vi "ESN_OnlineTraining.vi"(7 "Settings":cluster{"lamda":dbl, "Delta":dbl}={"lamda"=0.995, "Delta"=0.001}, 8 "error in (no error)":errorcluster, 9 "Desired Y(n+1)":dbl[](array[numeric]), 10 "input U(n+1)":dbl[](array[numeric]), 11 "ESN Status":T1) -> (0 "error out":errorcluster, 3 "ESN trained":T1)   [LabVIEW 2010]
uses:
  ESN_Network.ctl
  <vilib>/Analysis/Matrix/Datatypes/RealMatrix.ctl
  <vilib>/Analysis/Matrix/NI_Matrix.lvlib
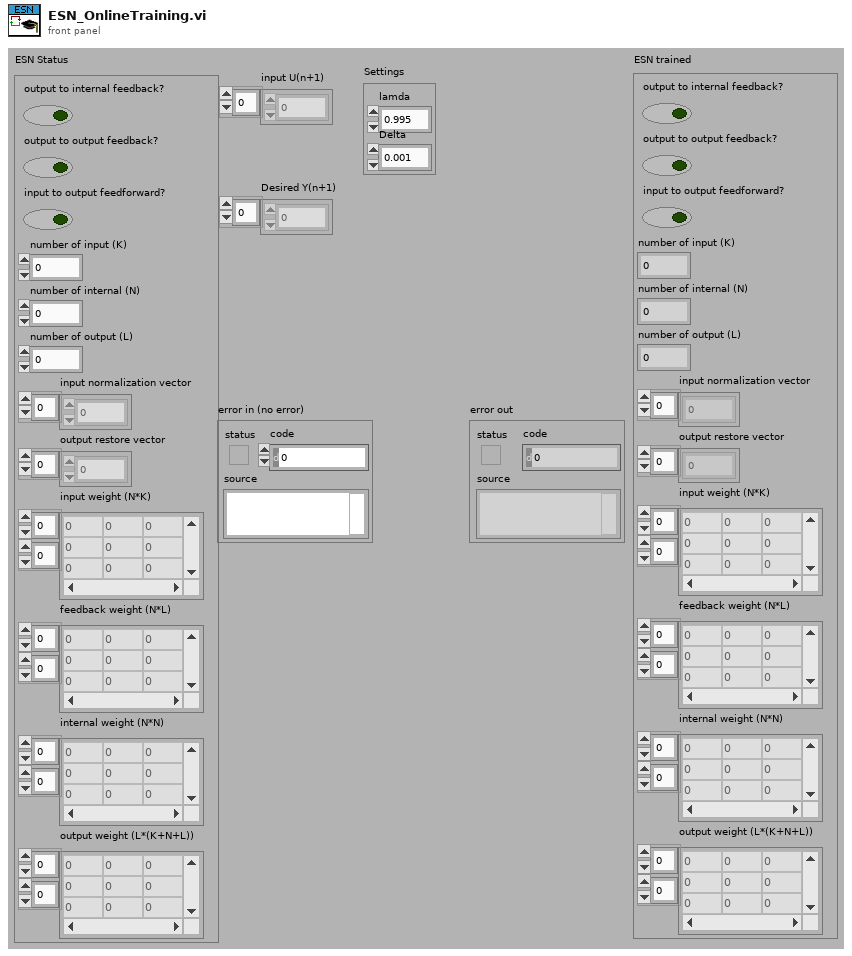
[diagram p1: front panel]
types:
  T1 = typedef "ESN_Network.ctl" = cluster{"output to internal feedback?":bool, "output to output feedback?":bool, "input to output feedforward?":bool, "number of input (K)":i32, "number of internal (N)":i32, "number of output (L)":i32, "input normalization vector":dbl[], "output restore vector":dbl[], "input weight (N*K)":T2, "feedback weight (N*L)":T2, "internal weight (N*N)":T2, "output weight (L*(K+N+L))":T2}
  T2 = typedef "NI_Matrix.lvlib/RealMatrix.ctl" = dbl[][]
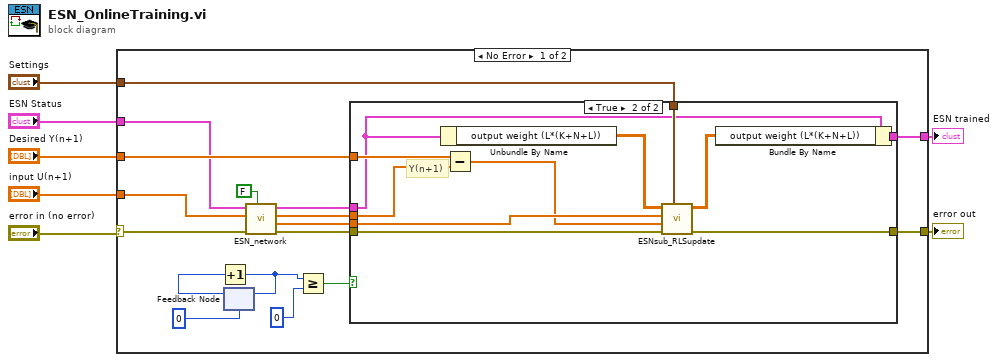
[diagram p0: block diagram]
diagram:
  n1 = case shown="No Error" "error in (no error)" {
    selector: "error in (no error)" -> [w19 w39]
    tunnel: "ESN Status" -> [w15 w38]
    tunnel: [w23 w38] -> w6
    tunnel: "Desired Y(n+1)" -> [w22 _]
    tunnel: "input U(n+1)" -> [w16 _]
    tunnel: "Settings" -> [w20 _]
    tunnel: [w17 w39] -> w1
    frame No Error {
      n2 = feedback #1(0) -> (w12:i32)
      n3 = Increment(x=w12) -> (x+1=w10:i32)
      n4 = feedback-in #1(w10) -> ()
      n5 = call "ESN_network.vi"("In train phase? (F)"=FALSE ("In train phase?"), "error in (no error)"=w19, "input"=w16, "ESN Status"=w15) -> ("error out"=w18:errorcluster, "State collection"=w21:dbl[], "output"=w14:dbl[], "ESN dup"=w13:T1)  [unwired: 4 in]
      n6 = Greater Or Equal?(x=w10, y=0) -> (x >= y?=w8:bool)
      n7 = case shown="True" w8 {
        tunnel: [w25 w37] -> w23
        tunnel: w22 -> [_ w36]
        tunnel: w21 -> [_ w33]
        tunnel: w20 -> [_ w31]
        tunnel: w18 -> [w26 w30]
        tunnel: [w26 w29] -> w17
        tunnel: w14 -> [_ w28]
        tunnel: w13 -> [w25 w27]
        frame False {
        }
        frame True {
          # "Y(n+1)"
          n8 = Unbundle By Name(w27) -> ("output weight (L*(K+N+L))"=w35:T2)
          n9 = Subtract(x=w36, y=w28) -> (x-y=w32:dbl[])
          n10 = call "ESNsub_RLSupdate.vi"("Settings"=w31, "error in (no error)"=w30, "e(n-1)"=w32, "X(n)"=w33, "W"=w35) -> ("error out"=w29:errorcluster, "Wn+1"=w34:T2)  [unwired: 5 in]
          n11 = Bundle By Name(cluster=w27, "output weight (L*(K+N+L))"=w34) -> (w37:T1)
        }
      }
    }
    frame Error {
    }
  }
  "ESN trained" <- w6
  "error out" <- w1
